vi "ReadResponse.vi"(8 "error in (no error)":errorcluster, 10 "Command":string="WX,PRG=0000,BLK=000,CharacterString=\"HelloWord\"", 11 "connection ID":refnum<k5>) -> (0 "error out":errorcluster, 1 "OK (Only RX Commands)":bool, 2 "Command Executed Correctly":bool, 3 "connection ID out":refnum<k5>, 4 "B":string, 5 "A":string)   [LabVIEW 2018]
panel:
  out "array":string[](array[string])
  out "Response String":string
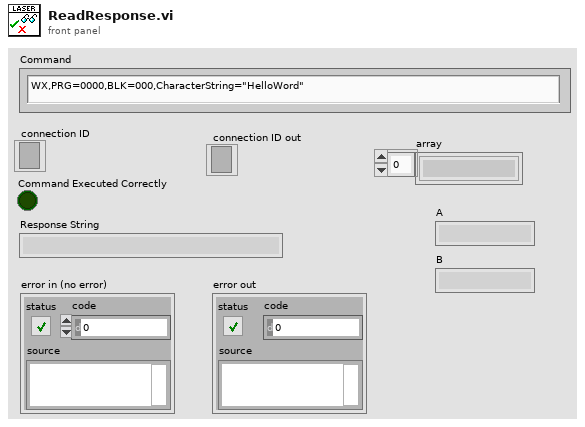
[diagram p1: front panel]
types:
  T1 = enum16{"Standard", "Buffered", "CRLF", "Immediate"}
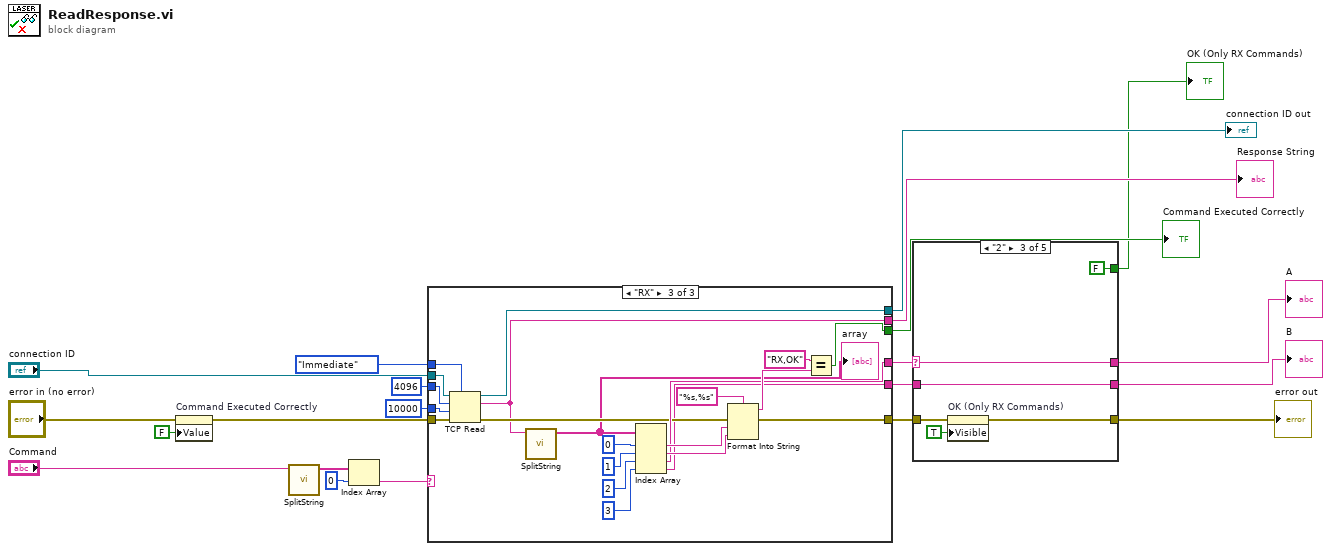
[diagram p0: block diagram]
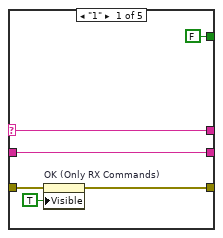
[diagram p2: hidden frame]
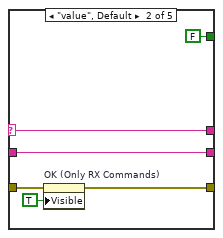
[diagram p3: hidden frame]
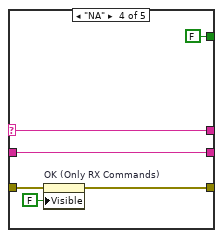
[diagram p4: hidden frame]
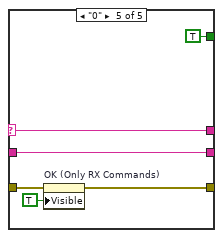
[diagram p5: hidden frame]
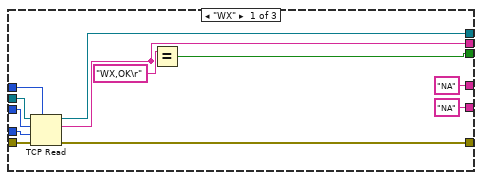
[diagram p6: hidden frame]
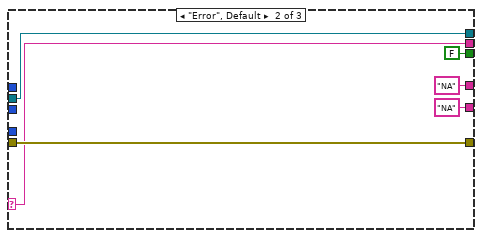
[diagram p7: hidden frame]
diagram:
  n1 = property on="Command Executed Correctly" class="Bool (strict)"(error in="error in (no error)", "Value"=FALSE ("command received")) -> (error out=w14:errorcluster)  [unwired: 1 in, 1 out]
  n2 = call "SplitString.vi"("Command"="Command") -> ("Array"=w6:string[])  [unwired: 10 in]
  n3 = Index Array(array=w6, index=0) -> (element=w4:string)
  n4 = case shown="\"RX\"" w4 {
    selector: w4 -> [_ w36 _]
    tunnel: w14 -> [w32 w37 w60]
    tunnel: [w23 w37 w44] -> w9
    tunnel: [w31 w36 w43] -> w12
    tunnel: T1."Immediate" ("mode (standard)") -> [w30 _ w59]
    tunnel: "connection ID" -> [w29 w39 w58]
    tunnel: 4096 ("bytes to read") -> [w28 _ w57]
    tunnel: 10000 ("timeout ms (25000)") -> [w27 _ w56]
    tunnel: [w26 w39 w55] -> w17
    tunnel: [w25 FALSE w54] -> w16
    tunnel: ["NA" ("String") "NA" ("String") w46] -> w11
    tunnel: ["NA" ("String") "NA" ("String") w40] -> w2
    frame "WX" {
      n5 = TCP Read(connection ID=w29, bytes to read=w28, error in (no error)=w32, 7:w30, 9:w27) -> (connection ID out=w26:refnum<k5>, data out=w31:string, error out=w23:errorcluster)
      n6 = Equal?(x="WX,OK\r", y=w31) -> (x = y?=w25:bool)
    }
    frame "Error", Default {
    }
    frame "RX" {
      n7 = TCP Read(connection ID=w58, bytes to read=w57, error in (no error)=w60, 7:w59, 9:w56) -> (connection ID out=w55:refnum<k5>, data out=w43:string, error out=w45:errorcluster)
      n8 = call "SplitString.vi"("Command"=w43) -> ("Array"=w42:string[])  [unwired: 10 in]
      "array" <- w42
      n9 = Index Array(array=w42, index #1=0 ("index"), index #2=1 ("index"), index #3=2 ("index"), index #4=3 ("index")) -> (element #1=w51:string, element #2=w50:string, element #3=w46:string, element #4=w40:string)
      n10 = Format Into String(format string="%s,%s", error in=w45, w51, w50) -> (resulting string=w48:string, error out=w44:errorcluster)  [unwired: 1 in]
      n11 = Equal?(x="RX,OK", y=w48) -> (x = y?=w54:bool)
    }
  }
  "Response String" <- w12
  "connection ID out" <- w17
  "Command Executed Correctly" <- w16
  n12 = case shown="\"2\"" w11 {
    selector: w11 -> [w63 w69 w75 w81 w87]
    tunnel: [FALSE ("OK?") FALSE ("OK?") FALSE ("OK?") FALSE ("OK?") TRUE ("OK?")] -> w10
    tunnel: w9 -> [w66 w72 w78 w84 w90]
    tunnel: [w65 w71 w77 w83 w89] -> w8
    tunnel: [w63 w69 w75 w81 w87] -> w3
    tunnel: w2 -> [w62 w68 w74 w80 w86]
    tunnel: [w62 w68 w74 w80 w86] -> w1
    frame "1" {
      n13 = property on="OK (Only RX Commands)" class="Bool (strict)"(error in=w66, "Visible"=TRUE) -> (error out=w65:errorcluster)  [unwired: 1 in, 1 out]
    }
    frame "value", Default {
      n14 = property on="OK (Only RX Commands)" class="Bool (strict)"(error in=w72, "Visible"=TRUE) -> (error out=w71:errorcluster)  [unwired: 1 in, 1 out]
    }
    frame "2" {
      n15 = property on="OK (Only RX Commands)" class="Bool (strict)"(error in=w78, "Visible"=TRUE) -> (error out=w77:errorcluster)  [unwired: 1 in, 1 out]
    }
    frame "NA" {
      n16 = property on="OK (Only RX Commands)" class="Bool (strict)"(error in=w84, "Visible"=FALSE) -> (error out=w83:errorcluster)  [unwired: 1 in, 1 out]
    }
    frame "0" {
      n17 = property on="OK (Only RX Commands)" class="Bool (strict)"(error in=w90, "Visible"=TRUE) -> (error out=w89:errorcluster)  [unwired: 1 in, 1 out]
    }
  }
  "error out" <- w8
  "OK (Only RX Commands)" <- w10
  "A" <- w3
  "B" <- w1
